vi "make1And2.vi"(8 "hight":dbl[](array[numeric])=[222.0, 143.0, 187.0], 9 "width":dbl[](array[numeric])=[1521.0, 47.0, 32.0], 10 "center":dbl[](array[numeric])=[85.0, 76.0, 75.0], 11 "MaxY":i32=222) -> (1 "min Y (2)":i32=137, 2 "emptyZArrayforreshape out":T1, 3 "min Y (1)":i32=137)   [LabVIEW 2020, in "MagAnalysis_Online.lvclass"]
uses:
  MagAnalysis_Online.lvclass
  emptyArray_TYpDEf.ctl
  emptyArrayCamX_TypDef.ctl
panel:
  out "Array":dbl[](array[numeric])
  out "x+y":dbl[](array[numeric])
  out "subarray 2":i32[](array[numeric])
  out "subarray":i32[](array[numeric])
  out "up":i32[][](array[numeric])=[[137, 1521], [146, 47], [147, 32]]
  out "low":i32[][](array[numeric])=[[85, 1521], [155, 47], [110, 32]]
  out "size":dbl[][](array[numeric])=[[222.0, 1521.0], [143.0, 47.0], [187.0, 32.0]]
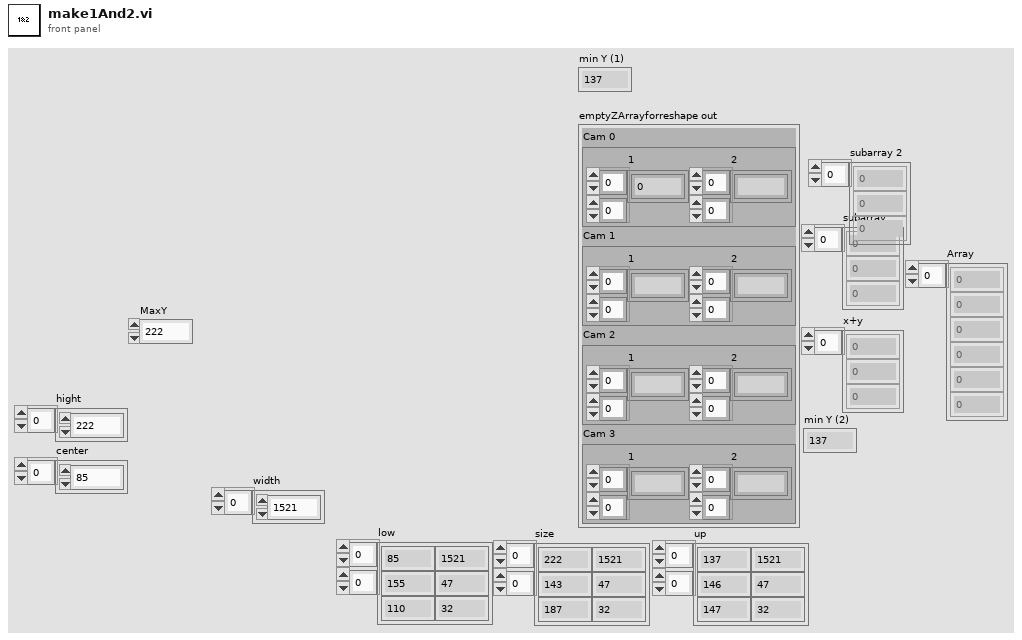
[diagram p1: front panel]
types:
  T1 = typedef "emptyArray_TYpDEf.ctl" = cluster{"Cam 0":T2, "Cam 1":T2, "Cam 2":T2, "Cam 3":T2}
  T2 = typedef "emptyArrayCamX_TypDef.ctl" = cluster{"1":dbl[][], "2":dbl[][]}
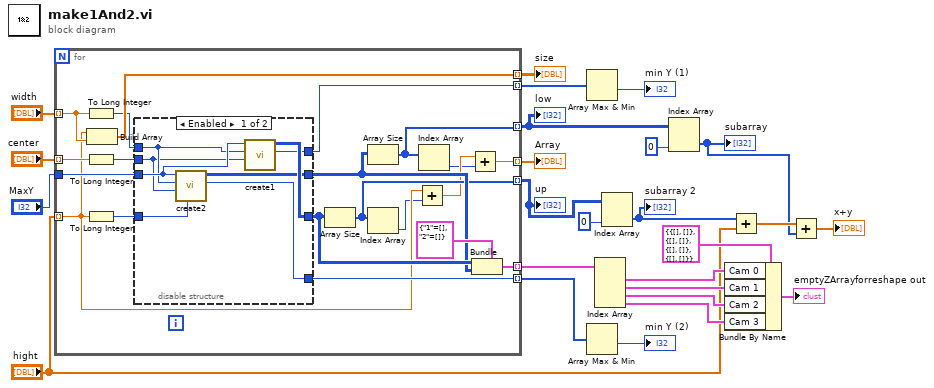
[diagram p0: block diagram]
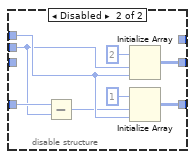
[diagram p2: hidden frame]
diagram:
  n1 = for {
    tunnel: "MaxY" -> [w45]
    tunnel: [w36] -> w22 mode=indexing
    tunnel: "width" -> [w41] mode=indexing
    tunnel: [w42] -> w21 mode=indexing
    tunnel: "hight" -> [w32] mode=indexing
    tunnel: "center" -> [w39] mode=indexing
    tunnel: [w40] -> w13 mode=indexing
    tunnel: [w33] -> w12 mode=indexing
    tunnel: [w34] -> w9 mode=indexing
    tunnel: [w35] -> w3 mode=indexing
    tunnel: [w30] -> w1 mode=indexing
    n2 = To Long Integer(number=w41) -> (32bit integer=w29:i32)
    n3 = To Long Integer(number=w39) -> (32bit integer=w44:i32)
    n4 = To Long Integer(number=w32) -> (32bit integer=w26:i32)
    n5 = Build Array(w32, w41) -> (w40:dbl[])
    n6 = disable-structure shown="Enabled" {
      disable-tunnel: w45 -> [w53 _]
      disable-tunnel: w29 -> [w52 w57]
      disable-tunnel: w44 -> [w51 w55]
      disable-tunnel: w26 -> [w50 w56]
      disable-tunnel: [w49 w60] -> w38
      disable-tunnel: [w48 w58] -> w37
      disable-tunnel: [w47 _] -> w36
      disable-tunnel: [w46 _] -> w35
      frame Enabled {
        n7 = call "create2.vi"("actual y size"=w50, "center"=w51, "X size"=w52, "max Y size"=w53) -> ("size"=w46:i32, "Array"=w48:i32[][])  [unwired: 6 in]
        n8 = call "create1.vi"("center"=w51, "X size"=w52, "max Y size"=w53) -> ("size"=w47:i32, "Array"=w49:i32[][])  [unwired: 7 in]
      }
      frame Disabled {
        n9 = Subtract(x=w56, y=w55) -> (x-y=w54:i32)
        n10 = Initialize Array(2 ("element"), w55, w57) -> (w58:i32[][])
        n11 = Initialize Array(1, w54, w57) -> (w60:i32[][])
      }
    }
    n12 = Array Size(array=w38) -> (size(s)=w34:i32[])
    n13 = Array Size(array=w37) -> (size(s)=w33:i32[])
    n14 = Index Array(array=w34) -> (element=w27:i32)  [unwired: 1 in]
    n15 = Add(x=w32, y=w27) -> (x+y=w31:dbl)
    n16 = Index Array(array=w33) -> (element=w28:i32)  [unwired: 1 in]
    n17 = Add(x=w31, y=w28) -> (x+y=w30:dbl)
    n18 = Bundle(cluster=T2 {"1"=[], "2"=[]} ("Cam 1"), "1"=w38, "2"=w37) -> (w42:T2)
  }
  "size" <- w13
  "low" <- w12
  "up" <- w9
  "Array" <- w1
  n19 = Array Max & Min(array=w22) -> (min value=→"min Y (1)":i32)  [unwired: 3 out]
  n20 = Array Max & Min(array=w3) -> (min value=→"min Y (2)":i32)  [unwired: 3 out]
  n21 = Index Array(array=w21) -> (element #1=w19:T2, element #2=w18:T2, element #3=w17:T2, element #4=w16:T2)  [unwired: 4 in]
  n22 = Index Array(array=w9, index (col)=0 ("disabled index (col)")) -> (element=w8:i32[])  [unwired: 1 in]
  "subarray 2" <- w8
  n23 = Index Array(array=w12, index (col)=0 ("disabled index (col)")) -> (element=w5:i32[])  [unwired: 1 in]
  "subarray" <- w5
  n24 = Bundle By Name(cluster=T1 {"Cam 0"={"1"=[], "2"=[]}, "Cam 1"={"1"=[], "2"=[]}, "Cam 2"={"1"=[], "2"=[]}, "Cam 3"={"1"=[], "2"=[]}} ("emptyZArrayforreshape in"), "Cam 0"=w19, "Cam 1"=w18, "Cam 2"=w17, "Cam 3"=w16) -> (→"emptyZArrayforreshape out":T1)
  n25 = Add(x=w8, y="hight") -> (x+y=w6:dbl[])
  n26 = Add(x=w6, y=w5) -> (x+y=→"x+y":dbl[])
